vi "Basic Example Demo.vi"() -> ()   [LabVIEW 2009]
uses:
  CAENComm.lvlib
panel:
  out "handle":i32
  out "log":string
  in  "read_mblt":bool
  in  "Address_mblt":u32 caption="Address:" format="%0x"
  in  "read":bool
  in  "write":bool
  in  "Size":u32(ring)=1 caption="Size:" items=["16 bit", "32 bit"]
  in  "Value":u32 caption="Value:" format="%0x"
  in  "Address":u32 caption="Address:" format="%0x"
  in  "clear_log":bool
  in  "get_info":bool
  in  "disconnet":bool
  in  "connect":bool
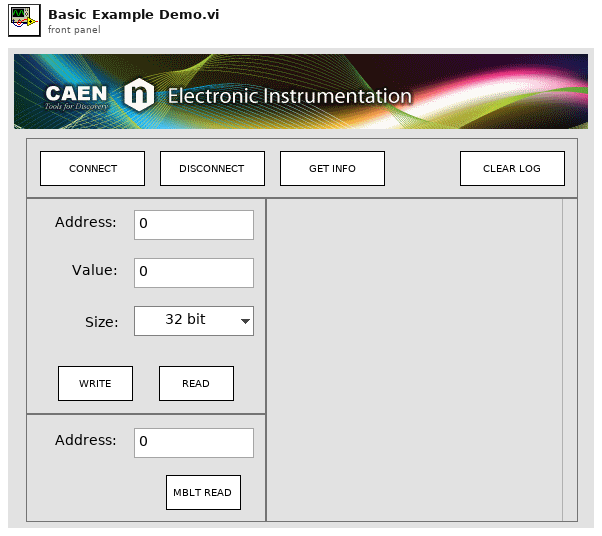
[diagram p1: front panel]
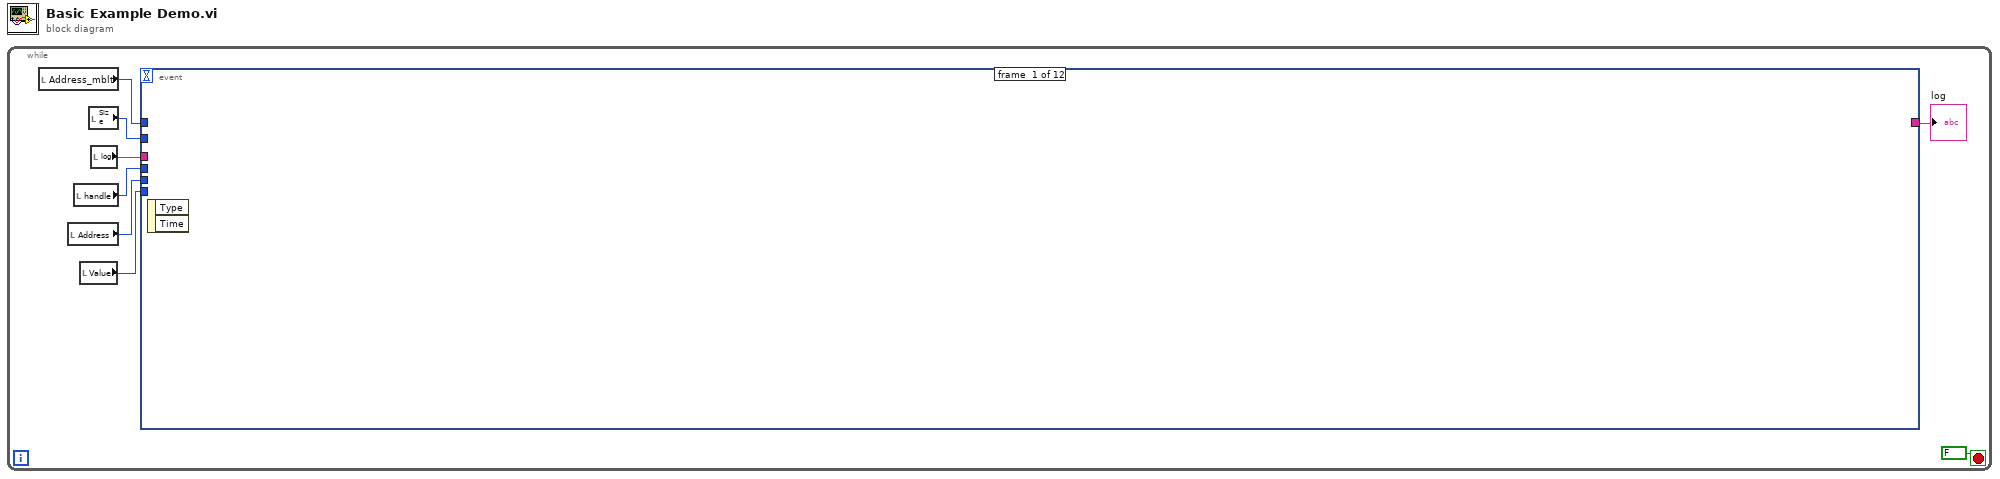
[diagram p0: block diagram]
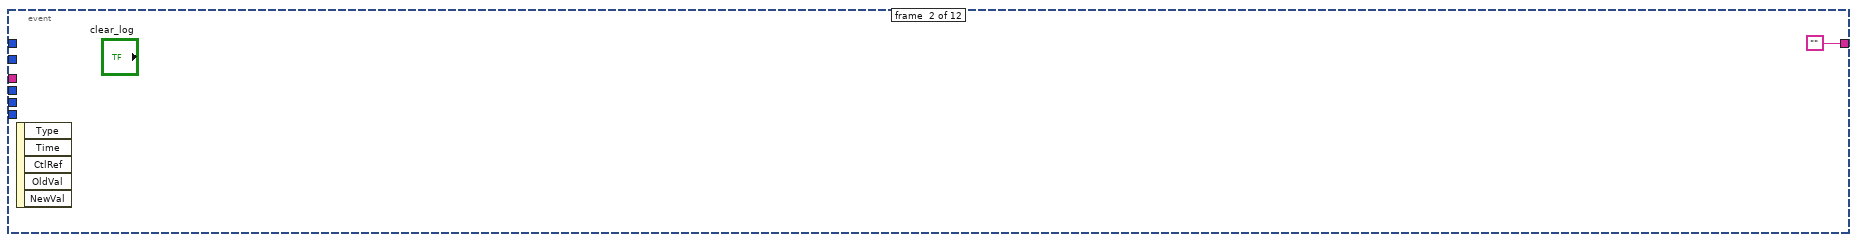
[diagram p2: hidden frame]
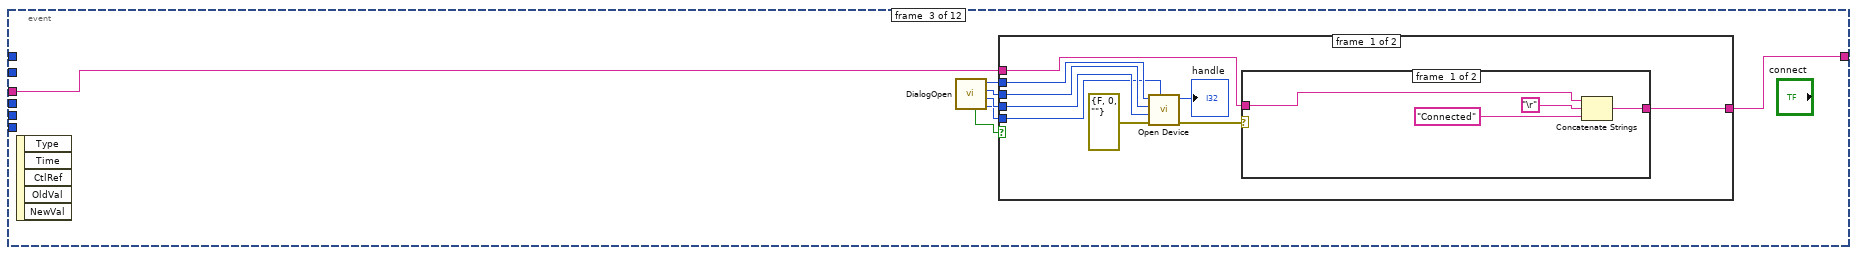
[diagram p3: hidden frame]
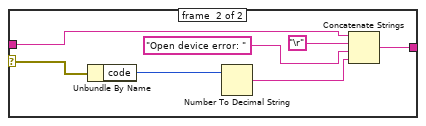
[diagram p4: hidden frame]
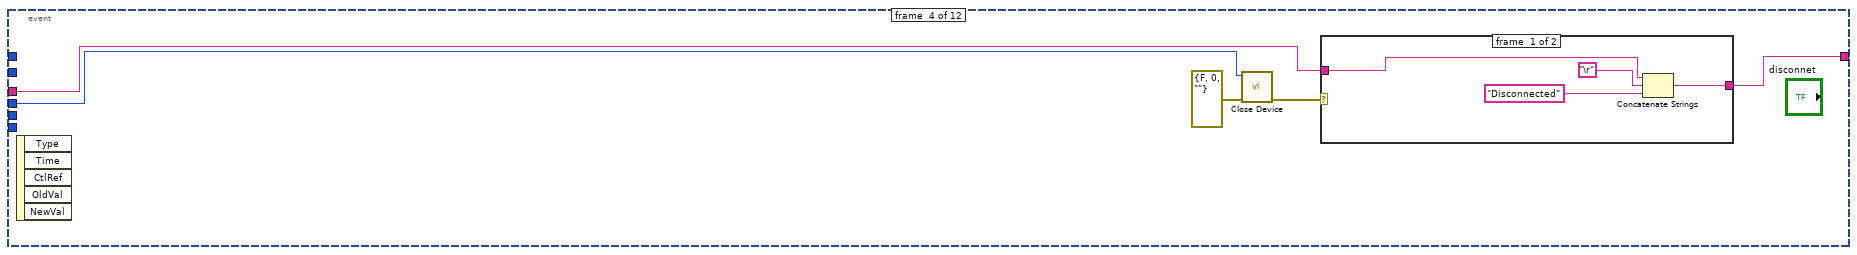
[diagram p6: hidden frame]
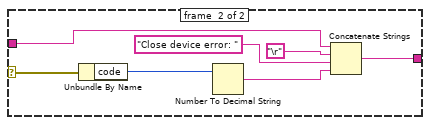
[diagram p7: hidden frame]
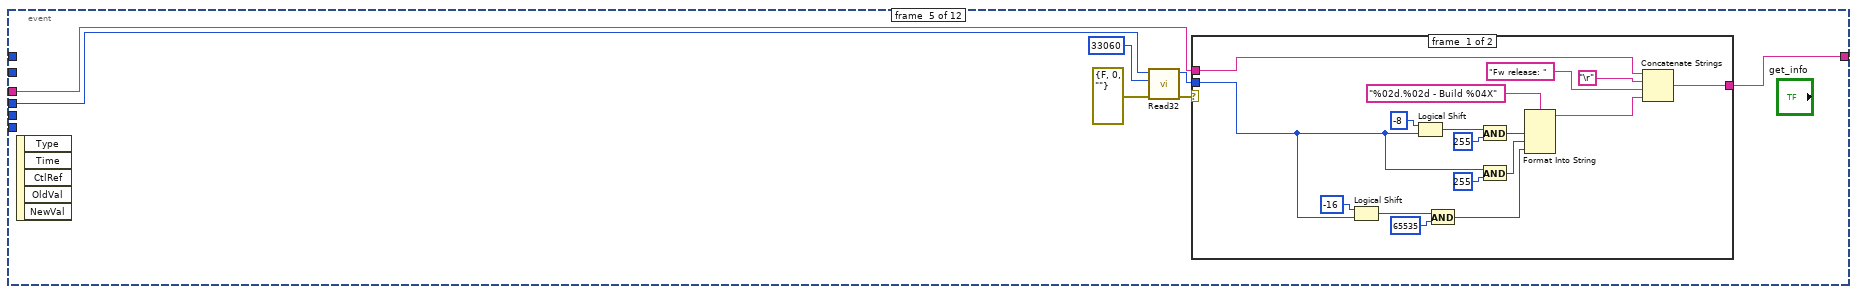
[diagram p8: hidden frame]
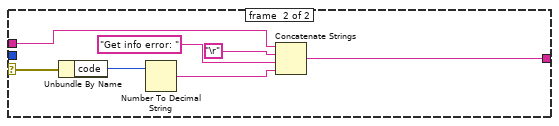
[diagram p9: hidden frame]
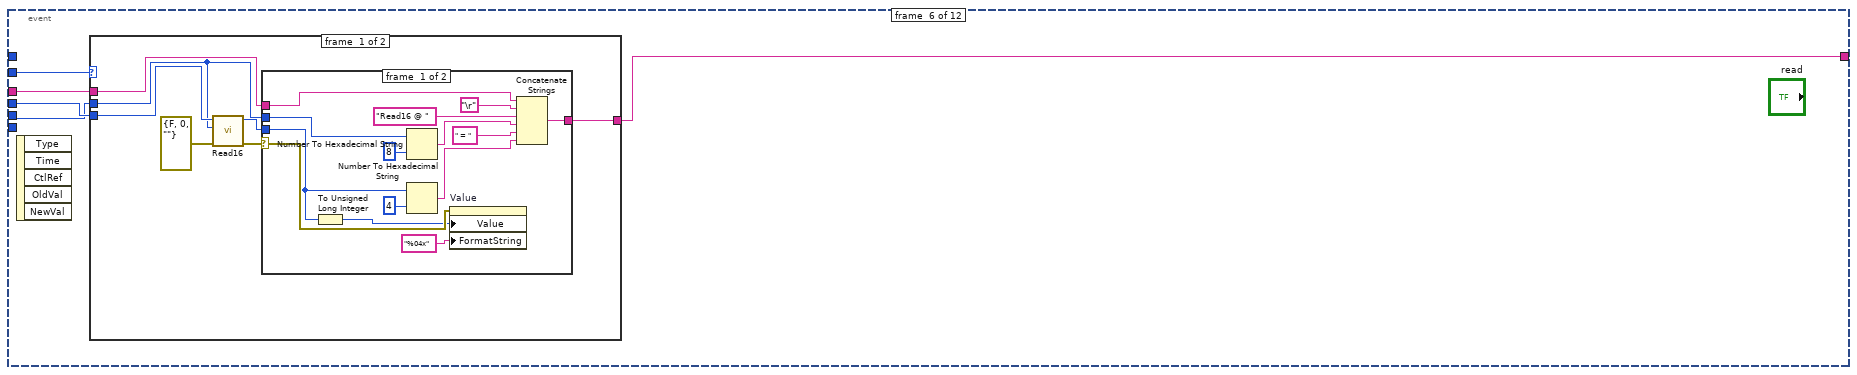
[diagram p10: hidden frame]
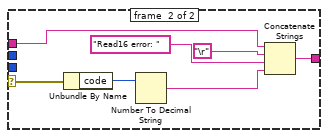
[diagram p11: hidden frame]
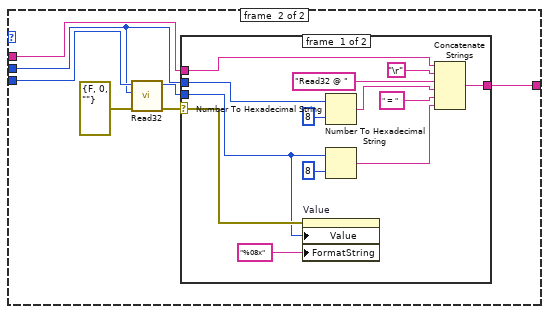
[diagram p12: hidden frame]
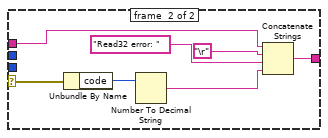
[diagram p13: hidden frame]
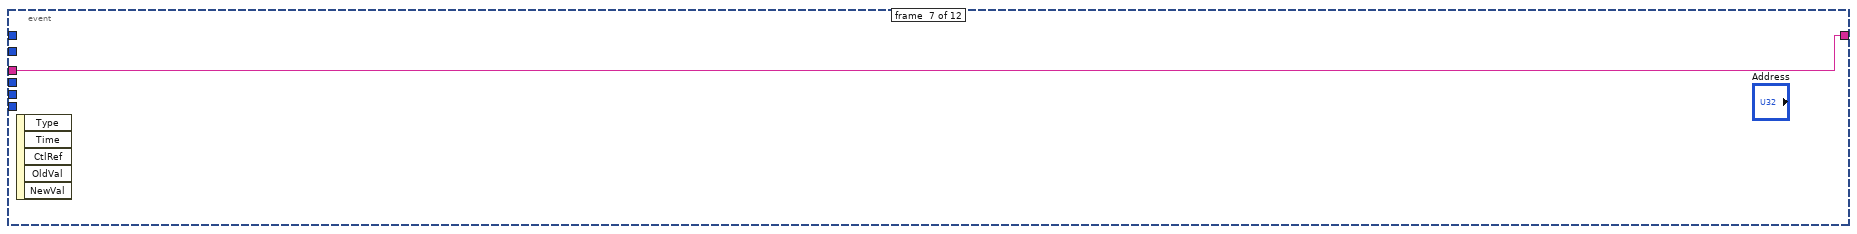
[diagram p14: hidden frame]
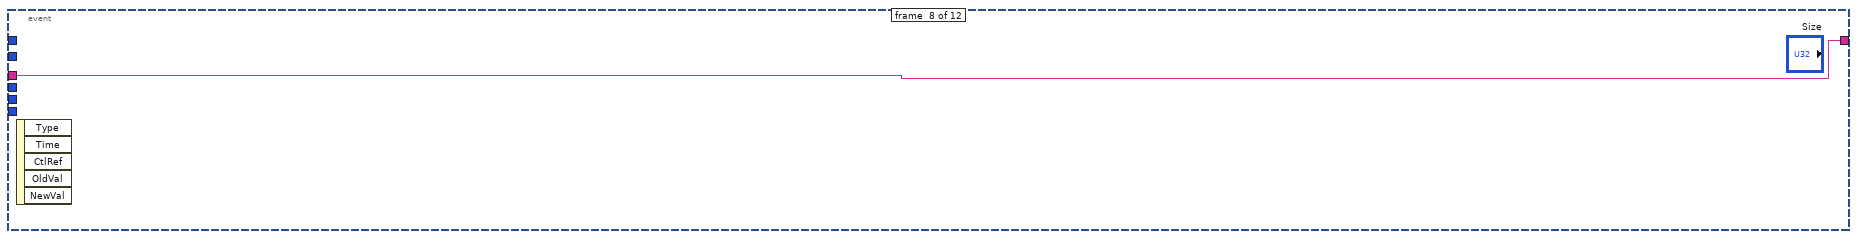
[diagram p15: hidden frame]
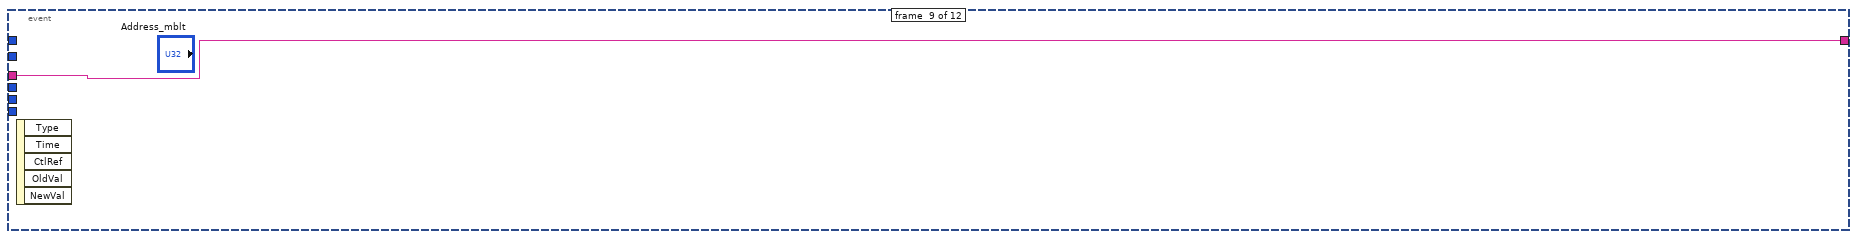
[diagram p16: hidden frame]
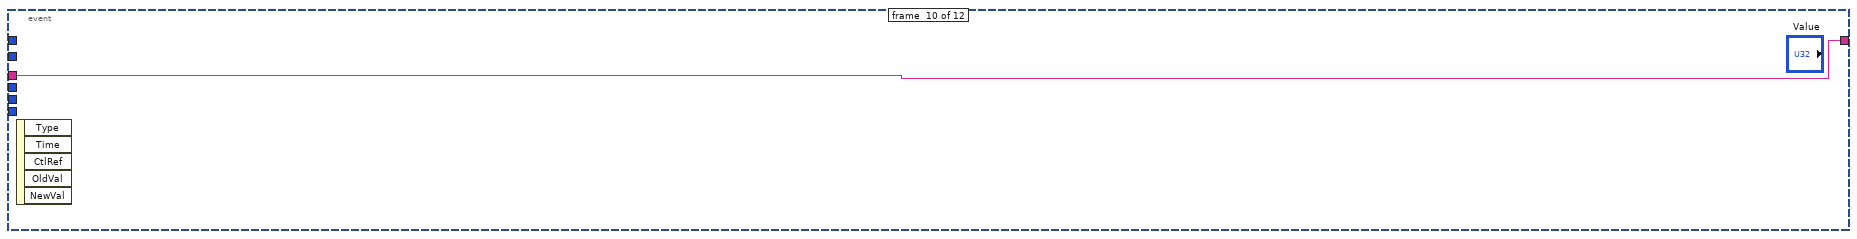
[diagram p17: hidden frame]
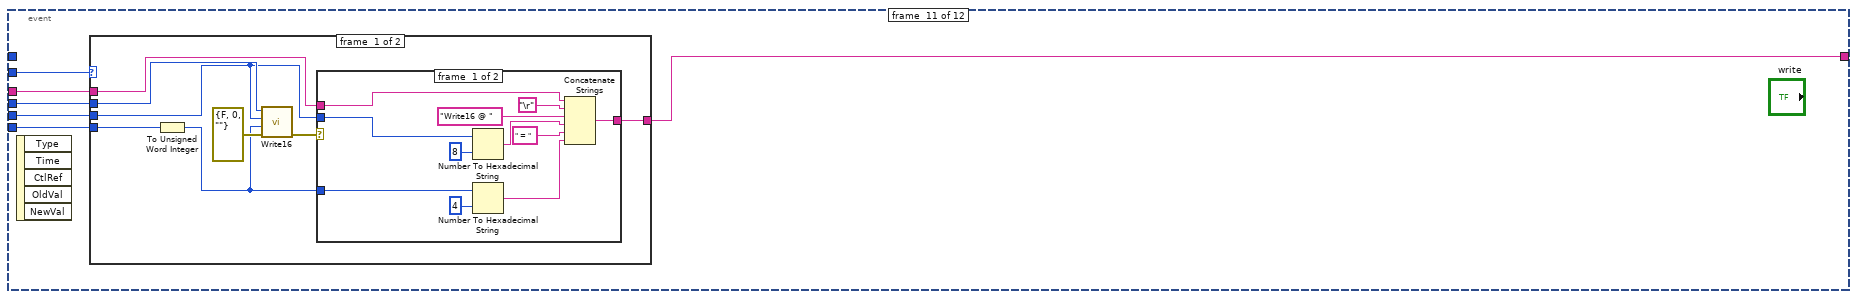
[diagram p18: hidden frame]
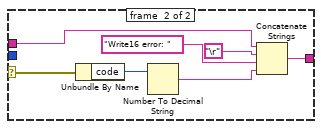
[diagram p19: hidden frame]
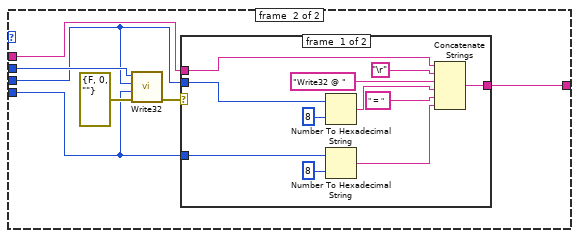
[diagram p20: hidden frame]
diagram:
  n1 = while {
    stop <- FALSE stop-if-true
    n2 = local read "Address_mblt"() -> (w2:u32)
    n3 = local read "Address"() -> (w4:u32)
    n4 = local read "handle"() -> (w6:i32)
    n5 = local read "Value"() -> (w1:u32)
    n6 = local read "Size"() -> (w3:u32)
    n7 = local read "log"() -> (w7:string)
    n8 = event shown="[11] \"read_mblt\": Value Change" {
      selector: _ -> [_ _ _ _ _ _ _ _ _ _ _ _]
      dyn-events: _ -> [_ _ _ _ _ _ _ _ _ _ _ _]
      timeout: _ -> [_ _ _ _ _ _ _ _ _ _ _ _]
      tunnel: [_ "" w11 w38 w59 w85 w145 w146 w147 w148 w150 w209] -> w8
      tunnel: w7 -> [_ _ w10 w39 w60 w86 w145 w146 w147 w148 w154 w217]
      tunnel: w6 -> [_ _ _ w42 w58 w89 _ _ _ _ w153 w219]
      tunnel: w3 -> [_ _ _ _ _ w88 _ _ _ _ w149 _]
      tunnel: w4 -> [_ _ _ _ _ w87 _ _ _ _ w152 _]
      tunnel: w1 -> [_ _ _ _ _ _ _ _ _ _ w151 _]
      tunnel: w2 -> [_ _ _ _ _ _ _ _ _ _ _ w218]
      event #0 {
        n9 = event-data() -> ()  [unwired: 1 in, 2 out]
      }
      event #1 {
        n10 = event-data() -> ()  [unwired: 1 in, 5 out]
      }
      event #2 {
        n11 = event-data() -> ()  [unwired: 1 in, 5 out]
        n12 = call "DialogOpen.vi"() -> ("VMEBaseAddress"=w13:u32, "ConetNode"=w14:i32, "LinkNum"=w15:i32, "LinkType"=w16:u32, "Cancelled?"=w12:bool)  [unwired: 7 in]
        n13 = case shown="False" w12 {
          tunnel: w16 -> [w25 _]
          tunnel: w15 -> [w24 _]
          tunnel: w14 -> [w23 _]
          tunnel: w13 -> [w22 _]
          tunnel: [w18 w37] -> w11
          tunnel: w10 -> [w17 w37]
          frame #0 {
            n14 = call "Open Device.vi"("VMEBaseAddress"=w22, "error in (no error)"=errorcluster {"status"=FALSE, "code"=0, "source"=""}, "ConetNode"=w23, "LinkNum"=w24, "LinkType"=w25) -> ("error out"=w19:errorcluster, "handle"=→"handle":i32)  [unwired: 5 in]
            n15 = case shown="No Error" w19 {
              selector: w19 -> [_ w33]
              tunnel: [w27 w34] -> w18
              tunnel: w17 -> [w26 w32]
              frame #0 {
                n16 = Concatenate Strings(w26, "\r", "Connected") -> (w27:string)
              }
              frame #1 {
                n17 = Unbundle By Name(w33) -> ("code"=w31:i32)
                n18 = Number To Decimal String(number=w31) -> (decimal integer string=w30:string)  [unwired: 1 in]
                n19 = Concatenate Strings(w32, "\r", "Open device error: ", w30) -> (w34:string)
              }
            }
          }
          frame #1 {
          }
        }
      }
      event #3 {
        n20 = event-data() -> ()  [unwired: 1 in, 5 out]
        n21 = call "Close Device.vi"("error in (no error)"=errorcluster {"status"=FALSE, "code"=0, "source"=""}, "handle"=w42) -> ("error out"=w40:errorcluster)  [unwired: 9 in]
        n22 = case shown="No Error" w40 {
          selector: w40 -> [_ w49]
          tunnel: w39 -> [w44 w48]
          tunnel: [w43 w47] -> w38
          frame #0 {
            n23 = Concatenate Strings(w44, "\r", "Disconnected") -> (w43:string)
          }
          frame #1 {
            n24 = Unbundle By Name(w49) -> ("code"=w51:i32)
            n25 = Number To Decimal String(number=w51) -> (decimal integer string=w50:string)  [unwired: 1 in]
            n26 = Concatenate Strings(w48, "\r", "Close device error: ", w50) -> (w47:string)
          }
        }
      }
      event #4 {
        n27 = event-data() -> ()  [unwired: 1 in, 5 out]
        n28 = call "Read32.vi"("error in (no error)"=errorcluster {"status"=FALSE, "code"=0, "source"=""}, "Address"=u32 33060, "handle"=w58) -> ("error out"=w55:errorcluster, "Data"=w54:u32)  [unwired: 7 in]
        n29 = case shown="No Error" w55 {
          selector: w55 -> [_ w79]
          tunnel: w60 -> [w76 w80]
          tunnel: [w75 w78] -> w59
          tunnel: w54 -> [w63 _]
          frame #0 {
            n30 = Logical Shift(y=i8 -16, x=w63) -> (x << y=w65:u32)
            n31 = Logical Shift(y=i8 -8, x=w63) -> (x << y=w68:u32)
            n32 = And(x=w65, y=u32 65535) -> (x .and. y?=w64:u32)
            n33 = And(x=w68, y=u32 255) -> (x .and. y?=w62:u32)
            n34 = And(x=w63, y=u32 255) -> (x .and. y?=w61:u32)
            n35 = Format Into String(format string="%02d.%02d - Build %04X", w62, w61, w64) -> (resulting string=w72:string)  [unwired: 2 in, 1 out]
            n36 = Concatenate Strings(w76, "\r", "Fw release: " ("string"), w72) -> (w75:string)
          }
          frame #1 {
            n37 = Unbundle By Name(w79) -> ("code"=w82:i32)
            n38 = Number To Decimal String(number=w82) -> (decimal integer string=w81:string)  [unwired: 1 in]
            n39 = Concatenate Strings(w80, "\r", "Get info error: ", w81) -> (w78:string)
          }
        }
      }
      event #5 {
        n40 = event-data() -> ()  [unwired: 1 in, 5 out]
        n41 = case shown="0" w88 {
          tunnel: w89 -> [w96 w120]
          tunnel: w87 -> [w91 w119]
          tunnel: w86 -> [w93 w124]
          tunnel: [w92 w123] -> w85
          frame #0 {
            n42 = call "Read16.vi"("error in (no error)"=errorcluster {"status"=FALSE, "code"=0, "source"=""}, "Address"=w91, "handle"=w96) -> ("error out"=w94:errorcluster, "Data"=w90:u16)  [unwired: 7 in]
            n43 = case shown="No Error" w94 {
              selector: w94 -> [w102 w111]
              tunnel: w93 -> [w108 w113]
              tunnel: [w103 w112] -> w92
              tunnel: w91 -> [w107 _]
              tunnel: w90 -> [w101 _]
              frame #0 {
                n44 = To Unsigned Long Integer(number=w101) -> (unsigned 32bit integer=w100:u32)
                n45 = Number To Hexadecimal String(1:i16 8 ("width (-)"), 2:w107) -> (0:w106:string)
                n46 = Number To Hexadecimal String(1:i16 4 ("width (-)"), 2:w101) -> (0:w104:string)
                n47 = property on="Value" class="DigNum (strict)"(error in=w102, "Value"=w100, "FormatString"="%04x" ("Format String")) -> ()  [unwired: 1 in, 2 out]
                n48 = Concatenate Strings(w108, "\r", "Read16 @ ", w106, " = " ("string"), w104) -> (w103:string)
              }
              frame #1 {
                n49 = Unbundle By Name(w111) -> ("code"=w115:i32)
                n50 = Number To Decimal String(number=w115) -> (decimal integer string=w114:string)  [unwired: 1 in]
                n51 = Concatenate Strings(w113, "\r", "Read16 error: ", w114) -> (w112:string)
              }
            }
          }
          frame #1 {
            n52 = call "Read32.vi"("error in (no error)"=errorcluster {"status"=FALSE, "code"=0, "source"=""}, "Address"=w119, "handle"=w120) -> ("error out"=w121:errorcluster, "Data"=w118:u32)  [unwired: 7 in]
            n53 = case shown="No Error" w121 {
              selector: w121 -> [w129 w138]
              tunnel: w124 -> [w135 w140]
              tunnel: [w130 w139] -> w123
              tunnel: w119 -> [w134 _]
              tunnel: w118 -> [w128 _]
              frame #0 {
                n54 = property on="Value" class="DigNum (strict)"(error in=w129, "Value"=w128, "FormatString"="%08x" ("Format String")) -> ()  [unwired: 1 in, 2 out]
                n55 = Number To Hexadecimal String(1:i16 8 ("width (-)"), 2:w134) -> (0:w133:string)
                n56 = Number To Hexadecimal String(1:i16 8 ("width (-)"), 2:w128) -> (0:w131:string)
                n57 = Concatenate Strings(w135, "\r", "Read32 @ ", w133, " = " ("string"), w131) -> (w130:string)
              }
              frame #1 {
                n58 = Unbundle By Name(w138) -> ("code"=w142:i32)
                n59 = Number To Decimal String(number=w142) -> (decimal integer string=w141:string)  [unwired: 1 in]
                n60 = Concatenate Strings(w140, "\r", "Read32 error: ", w141) -> (w139:string)
              }
            }
          }
        }
      }
      event #6 {
        n61 = event-data() -> ()  [unwired: 1 in, 5 out]
      }
      event #7 {
        n62 = event-data() -> ()  [unwired: 1 in, 5 out]
      }
      event #8 {
        n63 = event-data() -> ()  [unwired: 1 in, 5 out]
      }
      event #9 {
        n64 = event-data() -> ()  [unwired: 1 in, 5 out]
      }
      event #10 {
        n65 = event-data() -> ()  [unwired: 1 in, 5 out]
        n66 = case shown="1, Default" w149 {
          tunnel: w153 -> [w159 w184]
          tunnel: w152 -> [w158 w183]
          tunnel: w154 -> [w162 w187]
          tunnel: [w161 w186] -> w150
          tunnel: w151 -> [w156 w182]
          frame #0 {
            n67 = To Unsigned Word Integer(number=w156) -> (unsigned 16bit integer=w155:u16)
            n68 = call "Write16.vi"("error in (no error)"=errorcluster {"status"=FALSE, "code"=0, "source"=""}, "Data"=w155, "Address"=w158, "handle"=w159) -> ("error out"=w157:errorcluster)  [unwired: 7 in]
            n69 = case shown="No Error" w157 {
              selector: w157 -> [_ w174]
              tunnel: w162 -> [w171 w176]
              tunnel: [w166 w175] -> w161
              tunnel: w158 -> [w170 _]
              tunnel: w155 -> [w165 _]
              frame #0 {
                n70 = Number To Hexadecimal String(1:i16 8 ("width (-)"), 2:w170) -> (0:w169:string)
                n71 = Number To Hexadecimal String(1:i16 4 ("width (-)"), 2:w165) -> (0:w167:string)
                n72 = Concatenate Strings(w171, "\r", "Write16 @ ", w169, " = " ("string"), w167) -> (w166:string)
              }
              frame #1 {
                n73 = Unbundle By Name(w174) -> ("code"=w178:i32)
                n74 = Number To Decimal String(number=w178) -> (decimal integer string=w177:string)  [unwired: 1 in]
                n75 = Concatenate Strings(w176, "\r", "Write16 error: ", w177) -> (w175:string)
              }
            }
          }
          frame #1 {
            n76 = call "Write32.vi"("error in (no error)"=errorcluster {"status"=FALSE, "code"=0, "source"=""}, "Data"=w182, "Address"=w183, "handle"=w184) -> ("error out"=w181:errorcluster)  [unwired: 7 in]
            n77 = case shown="No Error" w181 {
              selector: w181 -> [_ w199]
              tunnel: w187 -> [w196 w201]
              tunnel: [w191 w200] -> w186
              tunnel: w183 -> [w195 _]
              tunnel: w182 -> [w190 _]
              frame #0 {
                n78 = Number To Hexadecimal String(1:i16 8 ("width (-)"), 2:w195) -> (0:w194:string)
                n79 = Number To Hexadecimal String(1:i16 8 ("width (-)"), 2:w190) -> (0:w192:string)
                n80 = Concatenate Strings(w196, "\r", "Write32 @ ", w194, " = " ("string"), w192) -> (w191:string)
              }
              frame #1 {
                n81 = Unbundle By Name(w199) -> ("code"=w203:i32)
                n82 = Number To Decimal String(number=w203) -> (decimal integer string=w202:string)  [unwired: 1 in]
                n83 = Concatenate Strings(w201, "\r", "Write32 error: ", w202) -> (w200:string)
              }
            }
          }
        }
      }
      event #11 {
        n84 = event-data() -> ()  [unwired: 1 in, 5 out]
        n85 = Concatenate Strings(w217, "\r", "-- Start of MBLT Read --" ("string")) -> (w221:string)
        n86 = property on="log" class="Str"(error in=errorcluster {"status"=FALSE, "code"=0, "source"=""} ("error in (no error)"), "Value"=w221) -> (error out=w208:errorcluster)  [unwired: 1 in, 1 out]
        n87 = property on="log" class="Str"(error in=w208) -> (error out=w207:errorcluster, "Value"=w206:string)  [unwired: 1 in, 1 out]
        n88 = while {
          shift-right: [w231] -> _
          shift-left: w207 -> [w230]
          tunnel: w219 -> [w236]
          tunnel: w218 -> [w235]
          tunnel: w206 -> [w232]
          shift-right: [w228] -> w210
          shift-left: 0 -> [w227]
          tunnel: [w226] -> w213
          stop <- w234 stop-if-true
          n89 = call "MBLT Read.vi"("error in (no error)"=w230, "BltSize"=2097152, "Address"=w235, "handle"=w236) -> ("error out"=w229:errorcluster, "nw"=w225:i32, "Buff"=w224:u32[])  [unwired: 5 in]
          n90 = Unbundle By Name(w229) -> ("code"=w233:i32)
          n91 = Not Equal To 0?(x=w233) -> (x != 0?=w234:bool)
          n92 = case shown="-13" w233 {
            selector: w233 -> [w238 _ _]
            tunnel: w232 -> [w240 w244 w261]
            tunnel: [w239 w246 w258] -> w226
            tunnel: w225 -> [_ w250 w263]
            tunnel: w224 -> [_ w251 w262]
            frame #0 {
              n93 = Number To Decimal String(number=w238) -> (decimal integer string=w241:string)  [unwired: 1 in]
              n94 = Concatenate Strings(w240, "\r", "MBLT Read error: ", w241) -> (w239:string)
            }
            frame #1 {
              w245 = "\r"
              n95 = for {
                N: w250 -> [_]
                tunnel: w251 -> [w255] mode=indexing
                shift-right: [w252] -> w248
                shift-left: "" -> [w257]
                n96 = Number To Hexadecimal String(1:i16 8 ("width (-)"), 2:w255) -> (0:w253:string)
                n97 = Concatenate Strings(w257, "\r", w253) -> (w252:string)
              }
              n98 = Concatenate Strings(w244, w245, w248, w245, "-- More --" ("string")) -> (w246:string)
            }
            frame #2 {
              n99 = for {
                N: w263 -> [_]
                tunnel: w262 -> [w268] mode=indexing
                shift-right: [w265] -> w259
                shift-left: "" -> [w270]
                n100 = Number To Hexadecimal String(1:i16 8 ("width (-)"), 2:w268) -> (0:w266:string)
                n101 = Concatenate Strings(w270, "\r", w266) -> (w265:string)
              }
              n102 = Concatenate Strings(w261, "\r", w259) -> (w258:string)
            }
          }
          n103 = Add(x=w227, y=w225) -> (x+y=w228:i32)
          n104 = property on="log" class="Str"(error in=w229, "Value"=w226) -> (error out=w231:errorcluster)  [unwired: 1 in, 1 out]
        }
        n105 = Number To Decimal String(number=w210) -> (decimal integer string=w214:string)  [unwired: 1 in]
        n106 = Concatenate Strings(w213, "\r", "-- End of MBLT Read: ", w214, " words --" ("string")) -> (w209:string)
      }
    }
    "log" <- w8
  }
